vi "gds_tx_init.vi"(8 "error in (no error)":errorcluster, 10 "HW parameters In":T3={"Device IP Address"="192.168.11.3", "Active Antenna"="TX1", "Carrier Frequency (Hz)"=915000000.0, "Gain (dB)"=10.0, "Generation Mode"=enum."continuous"} {"Gain (dB)" format="%.2f"; "Carrier Frequency (Hz)" format="%.2p"}, 11 "Modulation Parameters":T2) -> (0 "error out":errorcluster, 2 "HW parameters out":T3={"Device IP Address"="192.168.11.3", "Active Antenna"="RF1", "Carrier Frequency (Hz)"=2400000000.0, "Gain (dB)"=10.0, "Generation Mode"=enum."single shot"} {"Gain (dB)" format="%.2f"; "Carrier Frequency (Hz)" format="%.2p"}, 3 "Modulation Parameters Out":T2, 4 "coerced gain (dB)":dbl format="%#_6f", 6 "coerced carrier frequency (Hz)":dbl=100000.0 format="%#_6p")   [LabVIEW 2012]
uses:
  EE 497/LABS/SDR/control_type_defs.llb/tx_hw params.ctl
panel:
  in  "Configurations Out":T1(tab)
  in  "Configuration In":T1(tab)
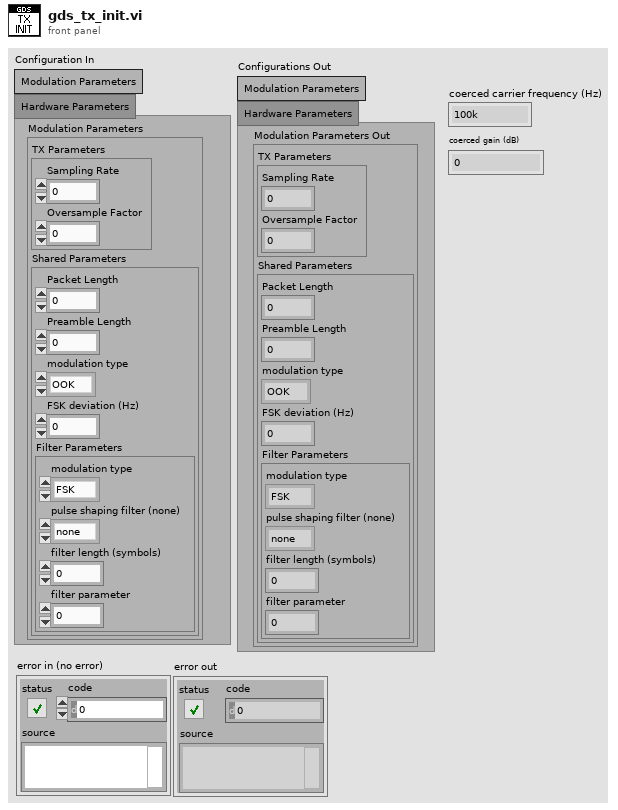
[diagram p1: front panel]
types:
  T1 = enum32{"Modulation Parameters", "Hardware Parameters"}
  T2 = cluster{"TX Parameters":cluster{"Sampling Rate":dbl, "Oversample Factor":i32}, "Shared Parameters":cluster{"Packet Length":i32, "Preamble Length":i32, "modulation type":enum16{"OOK", "FSK", "PSK", "QAM", "MSK", "PAM", "ASK", "CPM"}, "FSK deviation (Hz)":dbl, "Filter Parameters":cluster{"modulation type":enum16{"FSK", "PSK", "QAM", "MSK", "PAM", "ASK", "CPM"}, "pulse shaping filter (none)":enum16{"none", "Raised Cosine", "Root Raised Cos", "Gaussian"}, "filter length (symbols)":i32, "filter parameter":dbl}}}
  T3 = typedef "tx_hw params.ctl" = cluster{"Device IP Address":refnum<k15>, "Active Antenna":string, "Carrier Frequency (Hz)":dbl, "Gain (dB)":dbl, "Generation Mode":enum16{"single shot", "simulate", "continuous"}}
  T4 = cluster{"Sampling Rate":dbl, "Oversample Factor":i32}
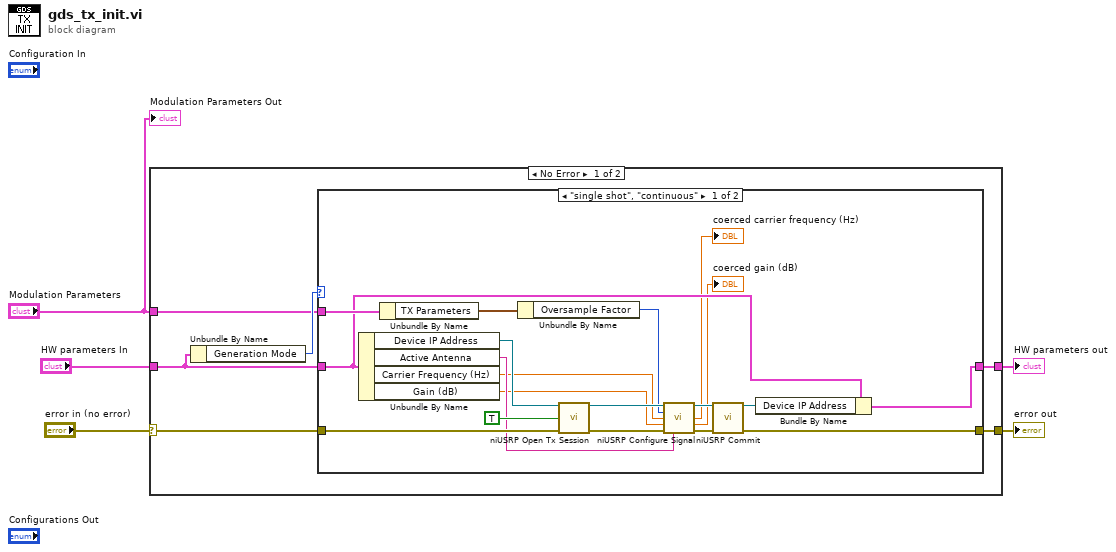
[diagram p0: block diagram]
diagram:
  n1 = case shown="No Error" "error in (no error)" {
    selector: "error in (no error)" -> [w8 w34]
    tunnel: [w7 w34] -> w4
    tunnel: [w10 w33] -> w3
    tunnel: "HW parameters In" -> [w9 w33]
    tunnel: "Modulation Parameters" -> [w6 _]
    frame No Error {
      n2 = Unbundle By Name(w9) -> ("Generation Mode"=w11:enum16{"single shot", "simulate", "continuous"})
      n3 = case shown="\"single shot\", \"continuous\"" w11 {
        tunnel: [w14 w32] -> w10
        tunnel: w9 -> [w15 w32]
        tunnel: w8 -> [w30 w31]
        tunnel: [w17 w31] -> w7
        tunnel: w6 -> [w29 _]
        frame "single shot", "continuous" {
          n4 = Unbundle By Name(w15) -> ("Device IP Address"=w27:refnum<k15>, "Active Antenna"=w24:string, "Carrier Frequency (Hz)"=w22:dbl, "Gain (dB)"=w21:dbl)
          n5 = Unbundle By Name(w29) -> ("TX Parameters"=w28:T4)
          n6 = Unbundle By Name(w28) -> ("Oversample Factor"=w20:i32)
          n7 = call <instrlib>:"niUSRP Open Tx Session.vi"("device names"=w27, "reset"=TRUE, "error in (no error)"=w30) -> ("session handle out"=w23:refnum<k15>, "error out"=w25:errorcluster)  [unwired: 11 in]
          n8 = call <instrlib>:"niUSRP Configure Signal.vi"("session handle"=w23, "IQ rate"=w20, "carrier frequency"=w22, "gain"=w21, "error in (no error)"=w25, "active antenna"=w24) -> ("session handle out"=w19:refnum<k15>, "coerced carrier frequency"=→"coerced carrier frequency (Hz)":dbl, "coerced gain"=→"coerced gain (dB)":dbl, "error out"=w18:errorcluster)  [unwired: 5 in, 1 out]
          n9 = call <instrlib>:"niUSRP Commit.vi"("session handle"=w19, "error in (no error)"=w18) -> ("session handle out"=w16:refnum<k15>, "error out"=w17:errorcluster)  [unwired: 12 in]
          n10 = Bundle By Name(cluster=w15, "Device IP Address"=w16) -> (w14:T3)
        }
        frame "simulate", Default {
        }
      }
    }
    frame Error {
    }
  }
  "error out" <- w4
  "HW parameters out" <- w3
  "Modulation Parameters Out" <- "Modulation Parameters"
